vi "Untitled 7 (SubVI).vi"(10 "Boolean":bool, 11 "Numeric":sgl) -> (0 "error out":errorcluster, 2 "timed out?\nBattery Potentiometer\nPotentiometer":bool, 3 "Battery Potentiometer\nPotentiometer (3202)":sgl)   [LabVIEW 2015]
uses:
  <vilib>/ErrorRing/Error Ring.xnode
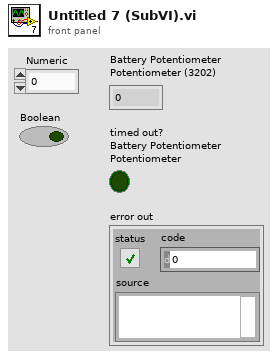
[diagram p1: front panel]
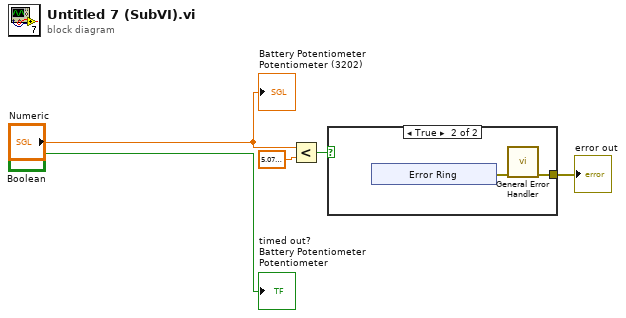
[diagram p0: block diagram]
diagram:
  n1 = Less?(x="Numeric", y=sgl 5.08) -> (x < y?=w5:bool)
  n2 = case shown="True" w5 {
    tunnel: [_ w7] -> w1
    frame False {
    }
    frame True {
      n3 = xnode "Error Ring"() -> ("error out"=w6:errorcluster)
      n4 = call <vilib>:"General Error Handler.vi"("error in (no error)"=w6) -> ("error out"=w7:errorcluster)  [unwired: 10 in, 4 out]
    }
  }
  "error out" <- w1
  "Battery Potentiometer\nPotentiometer (3202)" <- "Numeric"
  "timed out?\nBattery Potentiometer\nPotentiometer" <- "Boolean"
